vi "Initialize (SubVI).vi"() -> (0 "error out":errorcluster, 1 "Cluster":cluster{"ntf_ids":i32[], "ntfcrit_ids":i32[]}, 3 "token":string)   [LabVIEW 2020, in "Notification.lvlib"]
uses:
  Notification.lvlib
  <vilib>/Utility/config.llb/Read Key (String).vi
  <vilib>/Utility/config.llb/Read Key (I32).vi
  <vilib>/Utility/config.llb/NI_LVConfig.lvlib
panel:
  out "section names":string[](array[string])
  out "section":string
  out "section exists?":bool
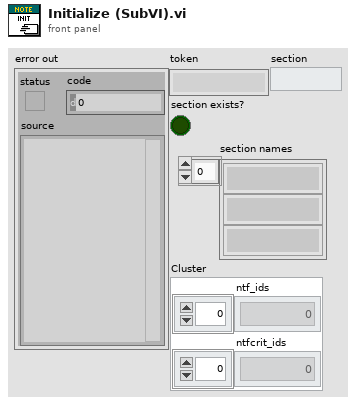
[diagram p1: front panel]
types:
  T1 = typedef "NI_LVConfig.lvlib/Config Data RefNum.ctl" = refnum<k1>
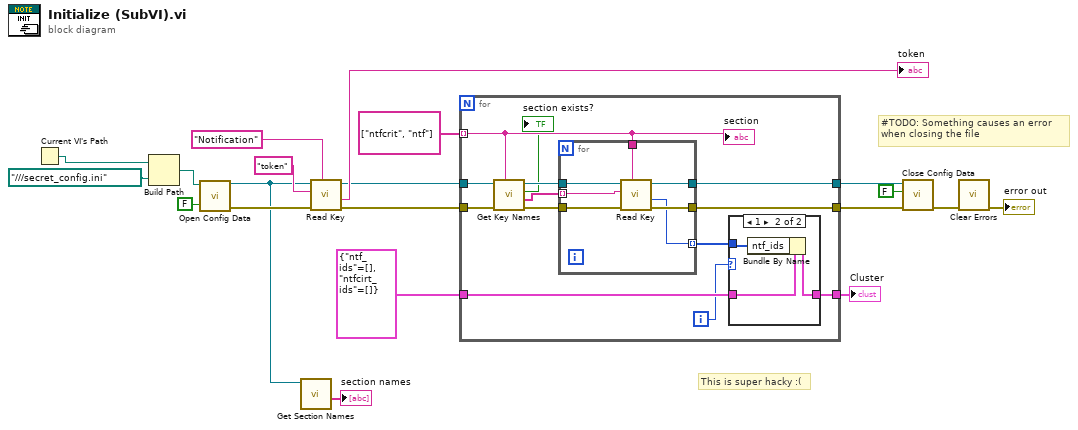
[diagram p0: block diagram]
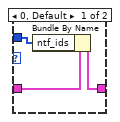
[diagram p2: hidden frame]
diagram:
  # "#TODO: Something causes an error\nwhen closing the file"
  # "This is super hacky :("
  n1 = Current VI's Path() -> (path=w17:path)
  n2 = Build Path(base path=w17, name or relative path=path "../../../secret_config.ini" ("configuration file path")) -> (appended path=w19:path)
  n3 = call <vilib>:"Open Config Data.vi"("create file if necessary (T)"=FALSE, "configuration file path"=w19) -> ("error out"=w15:errorcluster, "refnum"=w5:T1)  [unwired: 7 in, 1 out]
  n4 = call <vilib>:"Get Section Names.vi"("refnum"=w5) -> ("section names"=→"section names":string[])  [unwired: 8 in, 2 out]
  n5 = call-poly <vilib>:"Read Key.vi"("section"="Notification", "error in (no error)"=w15, "key"="token", "refnum"=w5) -> ("error out"=w9:errorcluster, "value"=→"token":string, "refnum out"=w8:T1)  [unwired: 4 in, 1 out]
  n6 = for {
    tunnel: string[] ["ntfcrit", "ntf"] -> [w26] mode=indexing
    tunnel: [w24] -> w2
    tunnel: cluster{"ntf_ids":i32[], "ntfcirt_ids":i32[]} {"ntf_ids"=[], "ntfcirt_ids"=[]} -> [w25]
    tunnel: w9 -> [w31]
    tunnel: [w33] -> w13
    tunnel: w8 -> [w29]
    tunnel: [w32] -> w12
    i -> [w23]
    n7 = call <vilib>:"Get Key Names.vi"("section"=w26, "error in (no error)"=w31, "refnum"=w29) -> ("error out"=w30:errorcluster, "key names"=w27:string[], "section exists?"=→"section exists?":bool, "refnum out"=w28:T1)  [unwired: 5 in]
    n8 = for {
      tunnel: w26 -> [w42]
      tunnel: w28 -> [w43]
      tunnel: [w45] -> w32
      tunnel: w27 -> [w41] mode=indexing
      tunnel: [w40] -> w22 mode=indexing
      tunnel: w30 -> [w44]
      tunnel: [w46] -> w33
      n9 = call-poly <vilib>:"Read Key.vi"("section"=w42, "error in (no error)"=w44, "key"=w41, "refnum"=w43) -> ("error out"=w46:errorcluster, "value"=w40:i32, "refnum out"=w45:T1)  [unwired: 4 in, 1 out]
    }
    n10 = case shown="1" w23 {
      tunnel: w25 -> [w36 w39]
      tunnel: [w35 w38] -> w24
      tunnel: w22 -> [w34 w37]
      frame 0, Default {
        n11 = Bundle By Name(cluster=w36, "ntf_ids"=w34) -> (w35:cluster{"ntf_ids":i32[], "ntfcirt_ids":i32[]})
      }
      frame 1 {
        n12 = Bundle By Name(cluster=w39, "ntf_ids"=w37) -> (w38:cluster{"ntf_ids":i32[], "ntfcirt_ids":i32[]})
      }
    }
    "section" <- w26
  }
  "Cluster" <- w2
  n13 = call <vilib>:"Close Config Data.vi"("error in (no error)"=w13, "write file if changed (T)"=FALSE, "refnum"=w12) -> ("error out"=w16:errorcluster)  [unwired: 7 in, 1 out]
  n14 = call <vilib>:"Clear Errors.vi"("error in (no error)"=w16) -> ("error out"=→"error out":errorcluster)  [unwired: 5 in, 1 out]
